vi "write_fifo.vi"(7 "pixel-to-host mode":T1, 8 "FIFO overflow in":bool, 9 "bitshift":i8, 10 "block index in":i32, 11 "values to be written":T2) -> (0 "FIFO overflow out":bool, 2 "block index out":i32, 3 "channels out":T2)   [LabVIEW 2011]
uses:
  typedefs/channels_array.ctl
  typedefs/pixel_to_host_enum.ctl
  <vilib>/rvi/interface/RandomDataEmulation/nirviRandomDataFPGAFIFO.vi
  <vilib>/rvi/interface/RandomDataEmulation/niFpgaRandomDataHandleErrors.vi
  <vilib>/rvi/DataTransferAndStorage/Container/XNode/niFpgaContainer.xnode
  <vilib>/rvi/interface/RandomDataEmulation/nirviRandomDataFpgaReadWriteTemplate.vi
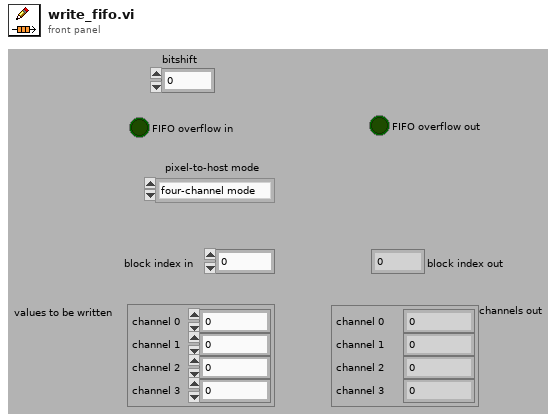
[diagram p1: front panel]
types:
  T1 = typedef "pixel_to_host_enum.ctl" = enum16{"four-channel mode", "two-channel mode"}
  T2 = typedef "channels_array.ctl" = cluster{"channel 0":u32, "channel 1":u32, "channel 2":u32, "channel 3":u32}
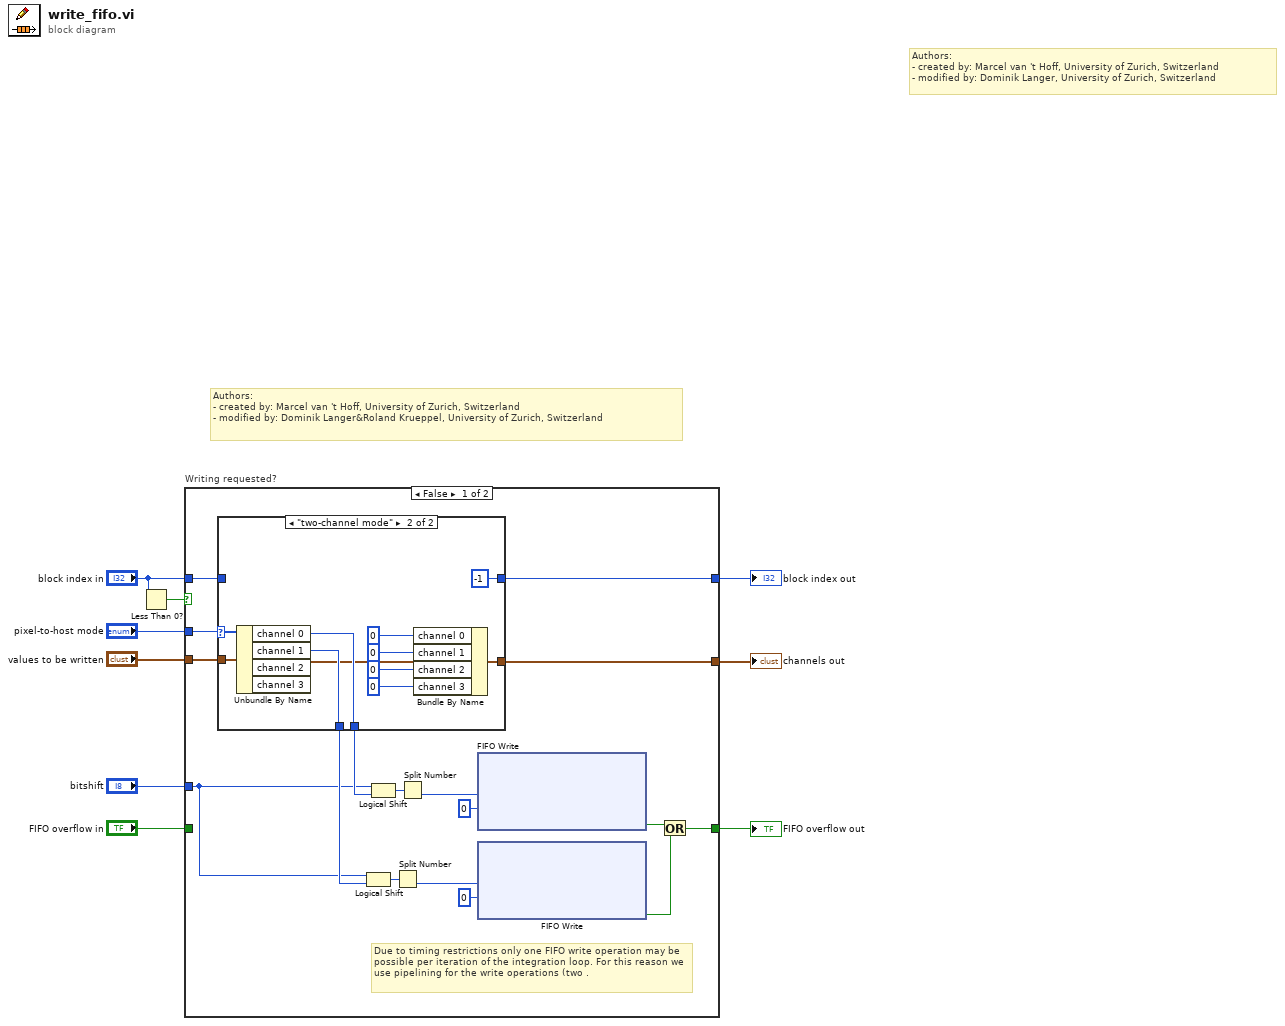
[diagram p0: block diagram]
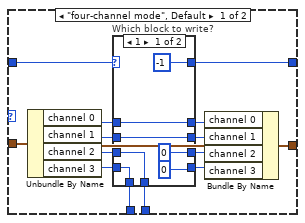
[diagram p2: hidden frame]
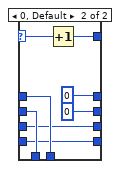
[diagram p3: hidden frame]
diagram:
  # "Authors: \n- created by: Marcel van 't Hoff, University of Zurich, Switzerland\n- modified by: Dominik Langer&Roland Krueppel, University of Zurich, Switzerland"
  # "Authors: \n- created by: Marcel van 't Hoff, University of Zurich, Switzerland\n- modified by: Dominik Langer, University of Zurich, Switzerland"
  n1 = Less Than 0?(x="block index in") -> (x < 0?=w5:bool)
  n2 = case "Writing requested?" shown="False" w5 {
    tunnel: [w21 w66] -> w6
    tunnel: [w18 w67] -> w9
    tunnel: "block index in" -> [w20 w67]
    tunnel: "values to be written" -> [w19 w66]
    tunnel: "FIFO overflow in" -> [_ w65]
    tunnel: [w22 w65] -> w3
    tunnel: "bitshift" -> [w13 _]
    tunnel: "pixel-to-host mode" -> [w10 _]
    frame False {
      # "Due to timing restrictions only one FIFO write operation may be possible per iteration of the integration loop. For this reason we use pipelining for the write operations (two ."
      n3 = case shown="\"two-channel mode\"" w10 {
        tunnel: [w30 w58] -> w21
        tunnel: w20 -> [w27 _]
        tunnel: w19 -> [w32 w57]
        tunnel: [w31 -1 ("block index in")] -> w18
        tunnel: [w29 w63] -> w14
        tunnel: [w28 w64] -> w17
        frame "four-channel mode", Default {
          n4 = Unbundle By Name(w32) -> ("channel 0"=w33:u32, "channel 1"=w34:u32, "channel 2"=w35:u32, "channel 3"=w36:u32)
          n5 = case "Which block to write?" shown="1" w27 {
            selector: w27 -> [_ w48]
            tunnel: [w47 w55] -> w28
            tunnel: w33 -> [w45 w55]
            tunnel: [w46 w54] -> w29
            tunnel: w34 -> [w44 w54]
            tunnel: w35 -> [w47 w53]
            tunnel: w36 -> [w46 w52]
            tunnel: [u32 0 ("channel 2") w53] -> w38
            tunnel: [u32 0 ("channel 3") w52] -> w37
            tunnel: [w45 u32 0 ("channel 0")] -> w39
            tunnel: [w44 u32 0 ("channel 1")] -> w40
            tunnel: [-1 ("block index in") w49] -> w31
            frame 1 {
            }
            frame 0, Default {
              n6 = Increment(x=w48) -> (x+1=w49:i32)
            }
          }
          n7 = Bundle By Name(cluster=w32, "channel 0"=w39, "channel 1"=w40, "channel 2"=w38, "channel 3"=w37) -> (w30:T2)
        }
        frame "two-channel mode" {
          n8 = Unbundle By Name(w57) -> ("channel 0"=w64:u32, "channel 1"=w63:u32)  [unwired: 2 out]
          n9 = Bundle By Name(cluster=w57, "channel 0"=u32 0, "channel 1"=u32 0, "channel 2"=u32 0 ("channel 0"), "channel 3"=u32 0 ("channel 1")) -> (w58:T2)
        }
      }
      n10 = Logical Shift(y=w13, x=w14) -> (x << y=w15:u32)
      n11 = Logical Shift(y=w13, x=w17) -> (x << y=w16:u32)
      n12 = Split Number(x=w15) -> (lo(x)=w11:u16)  [unwired: 1 out]
      n13 = Split Number(x=w16) -> (lo(x)=w12:u16)  [unwired: 1 out]
      n14 = xnode ("FIFO Write")("Element"=w12, "Timeout"=0) -> ("Timed Out?"=w23:bool)  [unwired: 1 in, 1 out]
      n15 = xnode ("FIFO Write")("Element"=w11, "Timeout"=0) -> ("Timed Out?"=w24:bool)  [unwired: 1 in, 1 out]
      n16 = Or(x=w23, y=w24) -> (x .or. y?=w22:bool)
    }
    frame True {
    }
  }
  "channels out" <- w6
  "block index out" <- w9
  "FIFO overflow out" <- w3
